vi "Teleop.vi"(10 "Match Info":T1={"Autonomous Elapsed Seconds"=0.0, "TeleOp Elapsed Seconds"=0.0, "Disabled Elapsed Seconds"=0.0, "Visited Autonomous"=FALSE, "Visited TeleOp"=FALSE, "Visited Disabled"=FALSE, "Autonomous Settings"={"Autonomous Style"=enum."Independent", "VI Refnum"=refnum}}, 11 "Call Context":T2) -> ()   [LabVIEW 2012]
doc: "This VI is called for each TeleOp packet received from the DS where the robot is not disabled. It is often used to read from the joysticks and update I/O or to update setpoints for timed control loops. It should complete and return within 20 milliseconds or it may miss DS packets."
uses:
  <vilib>/Rock Robotics/WPI/DriverStation/WPI_DriverStationDerivedRobotMode.ctl
  <vilib>/Rock Robotics/WPI/DriverStation/WPI_DriverStationMatch Info.ctl
  Robot Global Data.vi
  <vilib>/Rock Robotics/WPI/Joystick/WPI_JoystickGetSetRefNum.vi
panel:
  out "Numeric 2":dbl
  out "Numeric":dbl
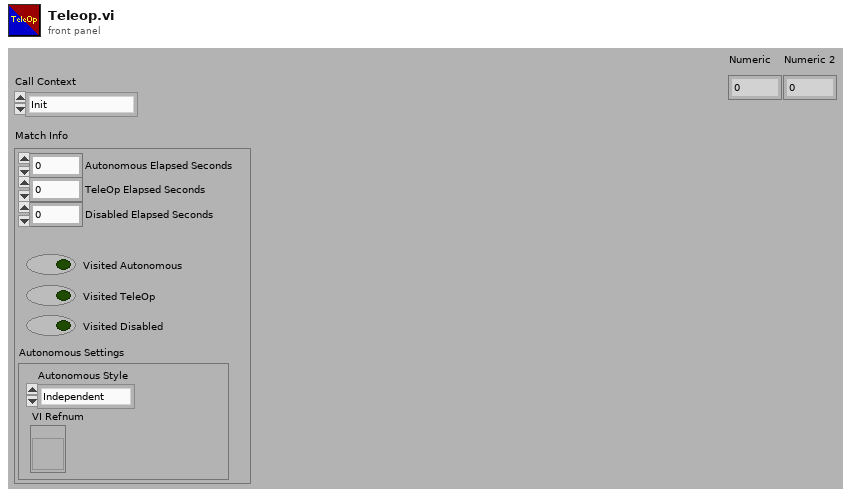
[diagram p1: front panel]
types:
  T1 = typedef "WPI_DriverStationMatch Info.ctl" = cluster{"Autonomous Elapsed Seconds":dbl, "TeleOp Elapsed Seconds":dbl, "Disabled Elapsed Seconds":dbl, "Visited Autonomous":bool, "Visited TeleOp":bool, "Visited Disabled":bool, "Autonomous Settings":cluster{"Autonomous Style":enum16{"Iterative", "Independent"}, "VI Refnum":refnum<vi>}}
  T2 = typedef "WPI_DriverStationDerivedRobotMode.ctl" = enum16{"Init", "Execute", "Stop"}
  T3 = typedef "WPI_JoystickDevRef.ctl" = cluster{"Device":T4}
  T4 = typedef "WPI_JoystickDeviceEnum.ctl" = enum16{"USB 1", "USB 2", "USB 3", "USB 4", "Kinect 1", "Kinect 2"}
  T5 = typedef "WPI_JoystickButtonState.ctl" = cluster{"Button 1":bool, "Button 2":bool, "Button 3":bool, "Button 4":bool, "Button 5":bool, "Button 6":bool, "Button 7":bool, "Button 8":bool, "Button 9":bool, "Button 10":bool, "Button 11":bool, "Button 12":bool}
  T6 = cluster{"axis 1 (x)":dbl, "axis 2 (y)":dbl, "axis 3 (throttle)":dbl, "axis 4":dbl, "axis 5":dbl, "axis 6":dbl}
  T7 = cluster{"Driver Station Digital Input (1-8)[0]":bool, "Driver Station Digital Input (1-8)[1]":bool, "Driver Station Digital Input (1-8)[2]":bool, "Driver Station Digital Input (1-8)[3]":bool, "Driver Station Digital Input (1-8)[4]":bool, "Driver Station Digital Input (1-8)[5]":bool, "Driver Station Digital Input (1-8)[6]":bool, "Driver Station Digital Input (1-8)[7]":bool, "Driver Station Digital Input (1-8)[8]":bool}
  T8 = cluster{"Shifting":cluster{"Right Servo High":dbl, "Right Servo Low":dbl, "Left Servo High":dbl, "Left Servo Low":dbl}, "Breaking":cluster{"Coast Position":dbl, "Break Position":dbl}}
  T9 = cluster{"Right Servo High":dbl, "Right Servo Low":dbl, "Left Servo High":dbl, "Left Servo Low":dbl}
  T10 = typedef "WPI_MotorControlDeviceRef.ctl" = cluster{"DeviceStatus":errorcluster, "Type":enum16{"PWM", "CAN"}, "PWM":cluster{"Digital Module":T11, "PWM Channel":T12, "DeadBand":T13}, "CAN":cluster{"Device Number":u8, "Control Mode":T14, "Semaphore":T15, "Max Vout":dbl}, "Invert":bool, "TransformRef":T16, "InvTransformRef":T16}
  T11 = typedef "FPGA_TypedefDigitalModule.ctl" = enum16{"Digital Module 1", "Digital Module 2"}
  T12 = typedef "FPGA_DIOPWMChannel.ctl" = enum8{"PWM 1", "PWM 2", "PWM 3", "PWM 4", "PWM 5", "PWM 6", "PWM 7", "PWM 8", "PWM 9", "PWM 10", "Invalid"}
  T13 = typedef "WPI_PWMDeadband.ctl" = cluster{"Name":string, "maxPositivePwm":i32, "minPositivePwm":i32, "centerPwm":i32, "maxNegativePwm":i32, "minNegativePwm":i32, "angularRange":u16}
  T14 = typedef "WPI_CANJaguar_ControlMode.ctl" = enum8{"Percent VBus", "Current", "Speed", "Position", "Voltage"}
  T15 = typedef "Semaphore RefNum" = refnum<k1>
  T16 = typedef "WPI_PWMTransform_ConPane.ctl" = refnum<vi>
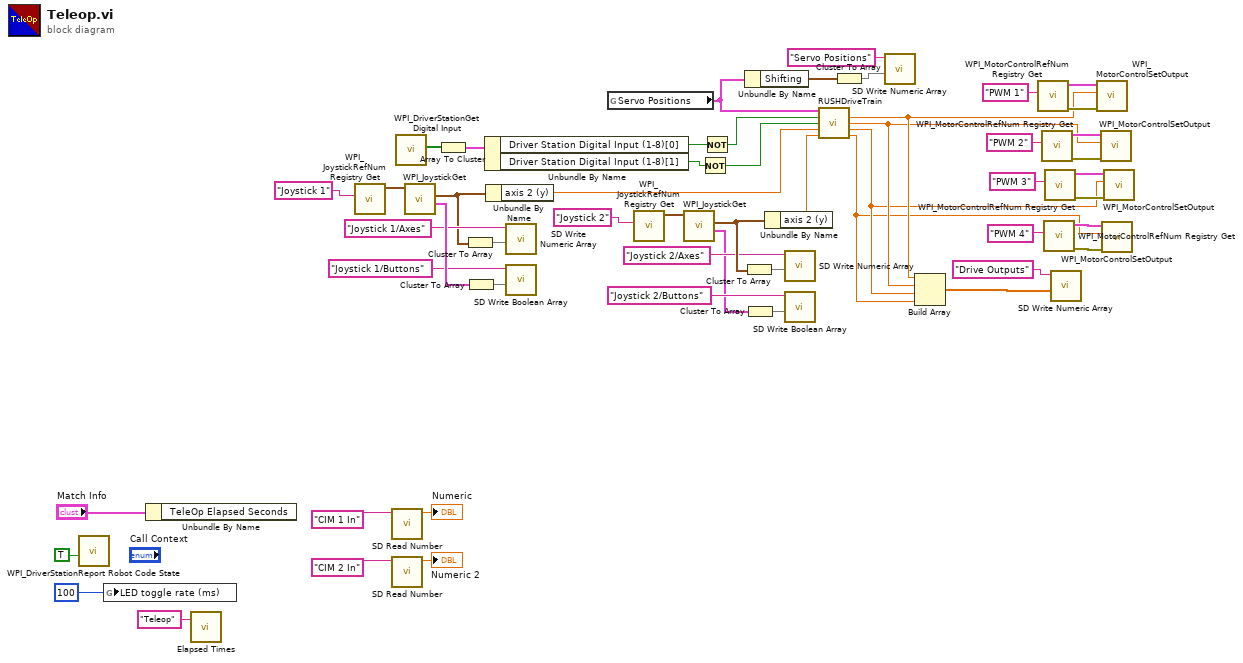
[diagram p0: block diagram]
diagram:
  n1 = call <vilib>:"WPI_DriverStationReport Robot Code State.vi"("TeleOp"=TRUE ("Autonomous")) -> ()  [unwired: 10 in, 1 out]
  n2 = global write "Robot Global Data.vi" "LED toggle rate (ms)"(u32 100 ("LED ms toggle rate")) -> ()
  n3 = Unbundle By Name("Match Info") -> ()  [unwired: 1 out]
  n4 = call "Elapsed Times.vi"("Call Name"="Teleop") -> ()  [unwired: 2 in, 1 out]
  n5 = call <vilib>:"WPI_JoystickRefNum Registry Get.vi"("refnum name"="Joystick 1") -> ("JoystickDevRef"=w52:T3)  [unwired: 1 in, 9 out]
  n6 = call <vilib>:"SD Read Number.vi"("Name"="CIM 1 In" ("refnum name")) -> ("Numeric"=→"Numeric":dbl)  [unwired: 8 in, 2 out]
  n7 = call <vilib>:"SD Read Number.vi"("Name"="CIM 2 In" ("refnum name")) -> ("Numeric"=→"Numeric 2":dbl)  [unwired: 8 in, 2 out]
  n8 = call <vilib>:"WPI_DriverStationGet Digital Input.vi"() -> ("Driver Station Digital Input (1-8)"=w33:bool[])  [unwired: 11 in]
  n9 = call <vilib>:"WPI_JoystickGet.vi"("JoystickDevRef"=w52) -> ("Buttons"=w49:T5, "Axes"=w42:T6)  [unwired: 1 in, 4 out]
  n10 = Array To Cluster(array=w33) -> (cluster=w32:T7)
  n11 = Cluster To Array(cluster=w42) -> (array=w46:dbl[])
  n12 = Cluster To Array(cluster=w49) -> (array=w48:bool[])
  n13 = Unbundle By Name(w32) -> ("Driver Station Digital Input (1-8)[0]"=w31:bool, "Driver Station Digital Input (1-8)[1]"=w30:bool)
  n14 = Unbundle By Name(w42) -> ("axis 2 (y)"=w27:dbl)
  n15 = call <vilib>:"SD Write Numeric Array.vi"("Numeric Array"=w46, "Name"="Joystick 1/Axes") -> ()  [unwired: 8 in, 2 out]
  n16 = call <vilib>:"SD Write Boolean Array.vi"("Boolean Array"=w48, "Name"="Joystick 1/Buttons") -> ()  [unwired: 8 in, 2 out]
  n17 = global read "Robot Global Data.vi" "Servo Positions"() -> (w25:T8)
  n18 = call <vilib>:"WPI_JoystickRefNum Registry Get.vi"("refnum name"="Joystick 2") -> ("JoystickDevRef"=w35:T3)  [unwired: 1 in, 9 out]
  n19 = call <vilib>:"WPI_JoystickGet.vi"("JoystickDevRef"=w35) -> ("Buttons"=w36:T5, "Axes"=w41:T6)  [unwired: 1 in, 4 out]
  n20 = Not(x=w30) -> (.not. x?=w28:bool)
  n21 = Not(x=w31) -> (.not. x?=w29:bool)
  n22 = Cluster To Array(cluster=w41) -> (array=w39:dbl[])
  n23 = Unbundle By Name(w25) -> ("Shifting"=w24:T9)
  n24 = Cluster To Array(cluster=w36) -> (array=w37:bool[])
  n25 = Unbundle By Name(w41) -> ("axis 2 (y)"=w26:dbl)
  n26 = call <vilib>:"SD Write Numeric Array.vi"("Numeric Array"=w39, "Name"="Joystick 2/Axes") -> ()  [unwired: 8 in, 2 out]
  n27 = call <vilib>:"SD Write Boolean Array.vi"("Boolean Array"=w37, "Name"="Joystick 2/Buttons") -> ()  [unwired: 8 in, 2 out]
  n28 = call "RUSHDriveTrain.vi"("Servo Positions"=w25, "Low Gear + Brake"=w29, "Low Gear"=w28, "LeftJoystick"=w27, "RightJoystick"=w26) -> ("Left Drive"=w7:dbl, "Right Drive"=w6:dbl, "Left Servo"=w5:dbl, "Right Servo"=w4:dbl)  [unwired: 6 in, 1 out]
  n29 = Cluster To Array(cluster=w24) -> (array=w23:dbl[])
  n30 = call <vilib>:"SD Write Numeric Array.vi"("Numeric Array"=w23, "Name"="Servo Positions") -> ()  [unwired: 8 in, 2 out]
  n31 = Build Array(w7, w6, w5, w4) -> (w21:dbl[])
  n32 = call <vilib>:"WPI_MotorControlRefNum Registry Get.vi"("refnum name"="PWM 1") -> ("error out"=w8:errorcluster, "MotorControlDevRef"=w9:T10)  [unwired: 9 in]
  n33 = call <vilib>:"WPI_MotorControlRefNum Registry Get.vi"("refnum name"="PWM 2") -> ("error out"=w13:errorcluster, "MotorControlDevRef"=w12:T10)  [unwired: 9 in]
  n34 = call <vilib>:"WPI_MotorControlRefNum Registry Get.vi"("refnum name"="PWM 4") -> ("error out"=w19:errorcluster, "MotorControlDevRef"=w18:T10)  [unwired: 9 in]
  n35 = call <vilib>:"WPI_MotorControlRefNum Registry Get.vi"("refnum name"="PWM 3") -> ("error out"=w14:errorcluster, "MotorControlDevRef"=w15:T10)  [unwired: 9 in]
  n36 = call <vilib>:"SD Write Numeric Array.vi"("Numeric Array"=w21, "Name"="Drive Outputs") -> ()  [unwired: 8 in, 2 out]
  n37 = call <vilib>:"WPI_MotorControlSetOutput.vi"("error in (no error)"=w8, "Output"=w7, "MotorControlDevRef"=w9) -> ()  [unwired: 6 in, 3 out]
  n38 = call <vilib>:"WPI_MotorControlSetOutput.vi"("error in (no error)"=w13, "Output"=w6, "MotorControlDevRef"=w12) -> ()  [unwired: 6 in, 3 out]
  n39 = call <vilib>:"WPI_MotorControlSetOutput.vi"("error in (no error)"=w19, "Output"=w4, "MotorControlDevRef"=w18) -> ()  [unwired: 6 in, 3 out]
  n40 = call <vilib>:"WPI_MotorControlSetOutput.vi"("error in (no error)"=w14, "Output"=w5, "MotorControlDevRef"=w15) -> ()  [unwired: 6 in, 3 out]
